vi "FileToArray(DBL).vi"(0 "path":path=path "C:/misc/LabVIEW/FILES/1D_array(col).psv", 3 "delimiter":string="|") -> (15 "data":dbl[][](array[numeric])=[[0.00033432], [0.0], [0.0], [3.432e-05]] format="%0.8f", 17 "# rows":i32, 19 "# cols":i32)   [LabVIEW 2014]
uses:
  <vilib>/Utility/file.llb/Read From Spreadsheet File (DBL).vi
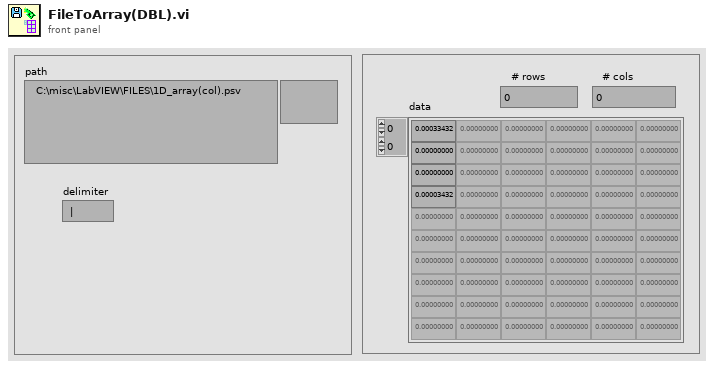
[diagram p1: front panel]
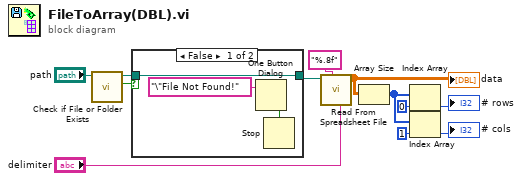
[diagram p0: block diagram]
diagram:
  n1 = call <vilib>:"Check if File or Folder Exists.vi"("path"="path") -> ("file or folder exists?"=w7:bool, "dup path"=w11:path)  [unwired: 8 in, 1 out]
  n2 = case shown="False" w7 {
    tunnel: w11 -> [w15 w16]
    tunnel: [w15 w16] -> w9
    frame False {
      n3 = One Button Dialog(message="\"File Not Found!") -> (true=w14:bool)  [unwired: 1 in]
      n4 = Stop(stop? (T)=w14) -> ()
    }
    frame True {
    }
  }
  n5 = call-poly <vilib>:"Read From Spreadsheet File.vi"("delimiter (\\t)"="delimiter", "format (%.3f)"="%.8f", "file path (dialog if empty)"=w9) -> ("all rows"=w6:dbl[][])  [unwired: 4 in, 4 out]
  "data" <- w6
  n6 = Array Size(array=w6) -> (size(s)=w2:i32[])
  n7 = Index Array(array=w2, index=0) -> (element=→"# rows":i32)
  n8 = Index Array(array=w2, index=1) -> (element=→"# cols":i32)
